vi "predict_signal_test_bench.vi"() -> ()   [LabVIEW 2020]
panel:
  out "Waveform Chart":cluster{"Slide":dbl, dbl}(graph)
  in  "Slide":dbl(slide) scale=0.0..10.0
  out "Numeric":i32
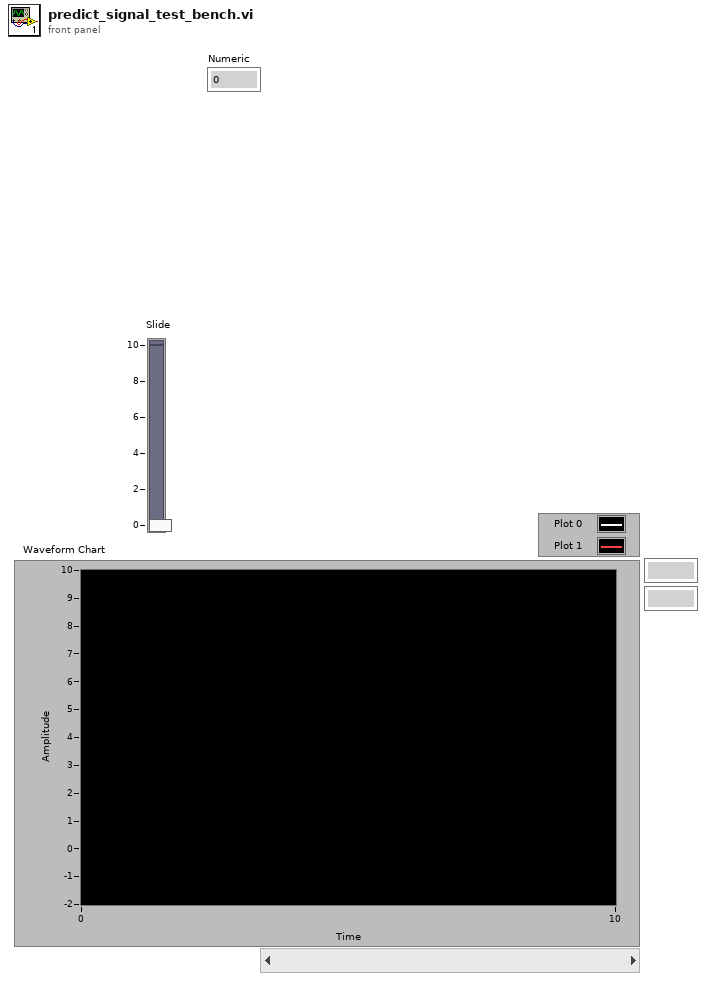
[diagram p1: front panel]
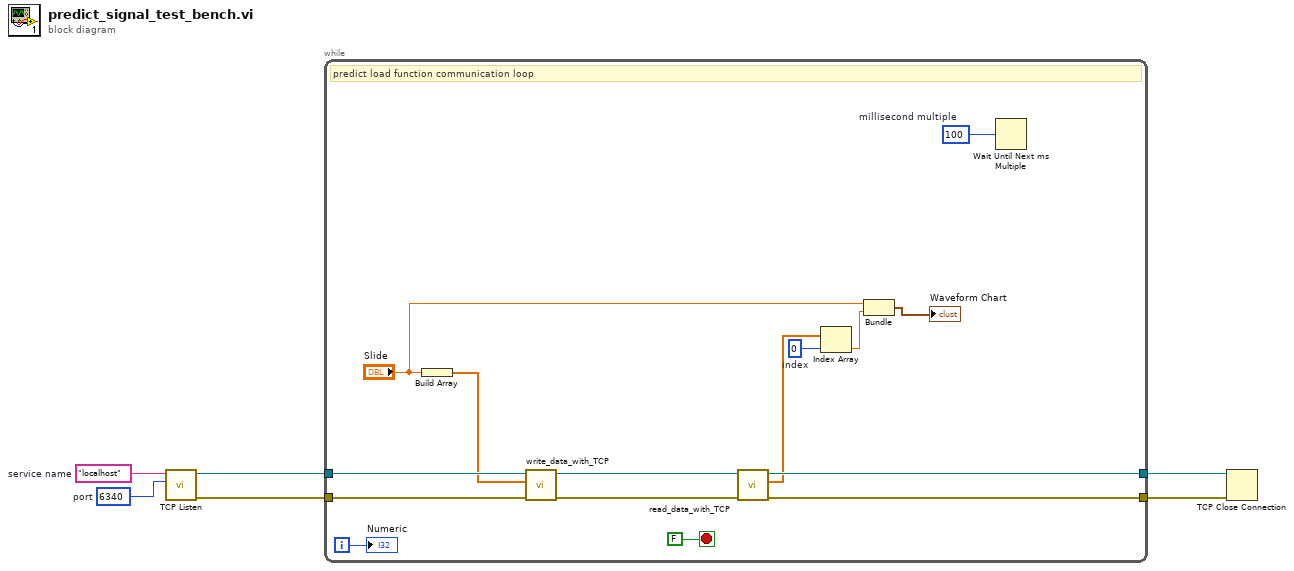
[diagram p0: block diagram]
diagram:
  w3 = u16 6340  # port
  w4 = "localhost"  # service name
  n1 = call <vilib>:"TCP Listen.vi"("port"=w3, "service name"=w4) -> ("error out"=w1:errorcluster, "connection ID"=w2:refnum<k5>)  [unwired: 5 in, 3 out]
  n2 = while {
    tunnel: w1 -> [w17]
    tunnel: w2 -> [w18]
    tunnel: [w15] -> w6
    tunnel: [w14] -> w5
    i -> [w20]
    stop <- FALSE stop-if-true
    w9 = 0  # index
    w12 = u32 100  # millisecond multiple
    # "predict load function communication loop"
    n3 = Build Array("Slide") -> (w13:dbl[])
    n4 = call "write_data_with_TCP.vi"("error_in"=w17, "data_in"=w13, "TCP_ref_in"=w18) -> ("error_out"=w19:errorcluster, "TCP_ref_out"=w16:refnum<k5>)  [unwired: 7 in]
    n5 = call "read_data_with_TCP.vi"("error_in"=w19, "TCP_ref_in"=w16) -> ("error_out"=w14:errorcluster, "data_out"=w10:dbl[], "TCP_ref_out"=w15:refnum<k5>)  [unwired: 7 in]
    n6 = Index Array(array=w10, index=w9) -> (element=w8:dbl)
    n7 = Bundle("Slide"="Slide", w8) -> (→"Waveform Chart":cluster{"Slide":dbl, dbl})  [unwired: 1 in]
    n8 = Wait Until Next ms Multiple(millisecond multiple=w12) -> ()  [unwired: 1 out]
    "Numeric" <- w20
  }
  n9 = TCP Close Connection(connection ID=w6, error in (no error)=w5) -> ()  [unwired: 1 in, 2 out]
